vi "Init.vi"(0 "reference in":refnum<class "Torque.lvclass">, 5 "error in (no error)":errorcluster) -> (14 "reference out":refnum<class "Torque.lvclass">, 19 "error out":errorcluster)   [LabVIEW 2013, in "Torque.lvclass"]
uses:
  Torque.lvclass
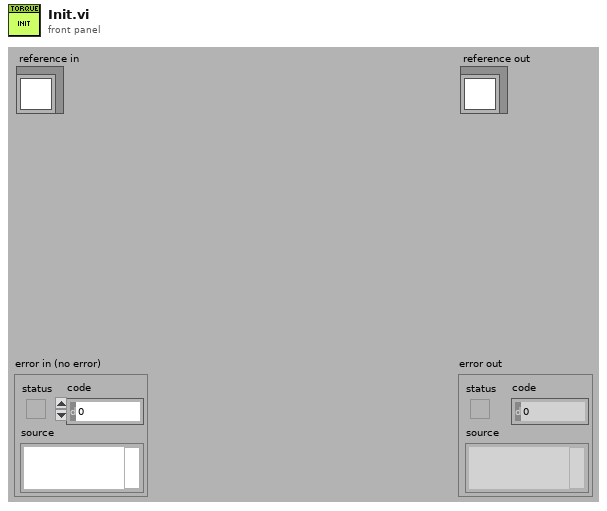
[diagram p1: front panel]
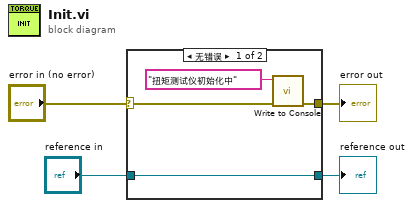
[diagram p0: block diagram]
diagram:
  n1 = case shown="无错误" "error in (no error)" {
    selector: "error in (no error)" -> [w7 w10]
    tunnel: [w5 w10] -> w3
    tunnel: [w8 w9] -> w1
    tunnel: "reference in" -> [w8 w9]
    frame No Error {
      n2 = call "Write to Console.vi"("error in (no error)"=w7, "Input"="扭矩测试仪初始化中") -> ("error out"=w5:errorcluster)  [unwired: 9 in]
    }
    frame Error {
    }
  }
  "error out" <- w3
  "reference out" <- w1
